vi "Set DDS Burst Style.vi"(10 "style":i32, 11 "channel_index":u8) -> ()   [LabVIEW 2021, in "vmmso.lvlib"]
doc: "DLL_API void WINAPI SetDDSBurstStyle(unsigned char channel_index, int style);"
uses:
  vmmso.lvlib
  vmmso.dll
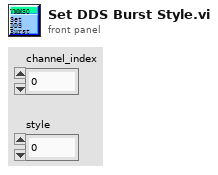
[diagram p1: front panel]
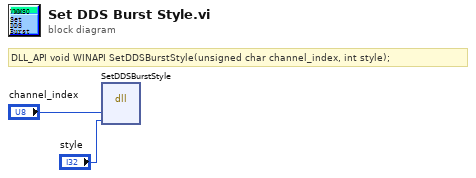
[diagram p0: block diagram]
diagram:
  # "DLL_API void WINAPI SetDDSBurstStyle(unsigned char channel_index, int style);"
  n1 = dll-call lib="D:/labviewdemo/LabviewDemo 21/vmmso/vmmso.*" fn="SetDDSBurstStyle"("channel_index"="channel_index", "style"="style") -> ()  [unwired: 6 in, 2 out]
